vi "Capture.vi"(0 "Victim ID":i32, 1 "Attacker ID":i32) -> ()   [LabVIEW 2025]
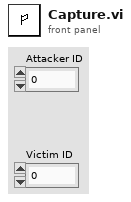
[diagram p1: front panel]
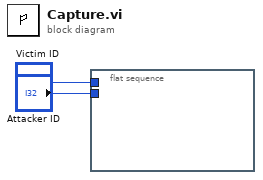
[diagram p0: block diagram]
diagram:
  n1 = flat-sequence {
    tunnel: "Victim ID" -> [_]
    tunnel: "Attacker ID" -> [_]
    frame #0 {
    }
  }
